vi "Number_2_string.vi"(1 "precision":string, 2 "number":dbl format="%.5f") -> (0 "String":string)   [LabVIEW 2020]
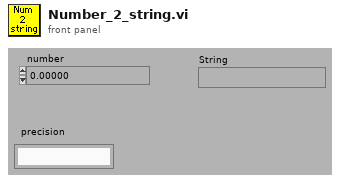
[diagram p1: front panel]
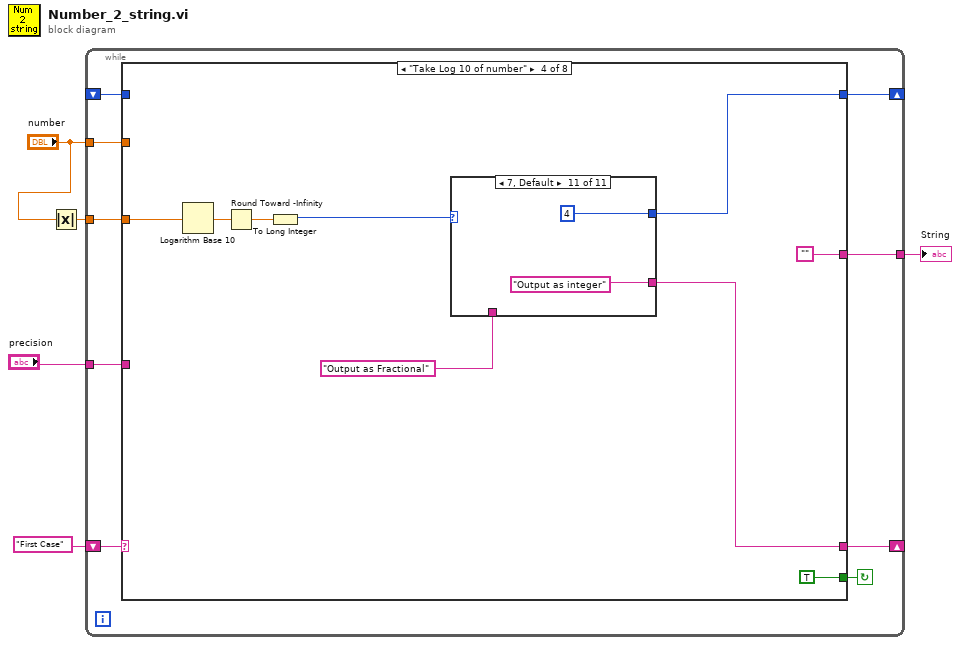
[diagram p0: block diagram]
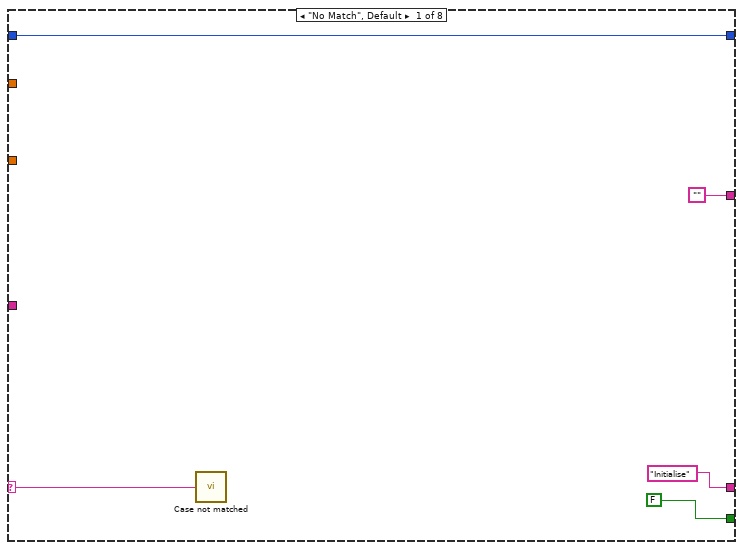
[diagram p2: hidden frame]
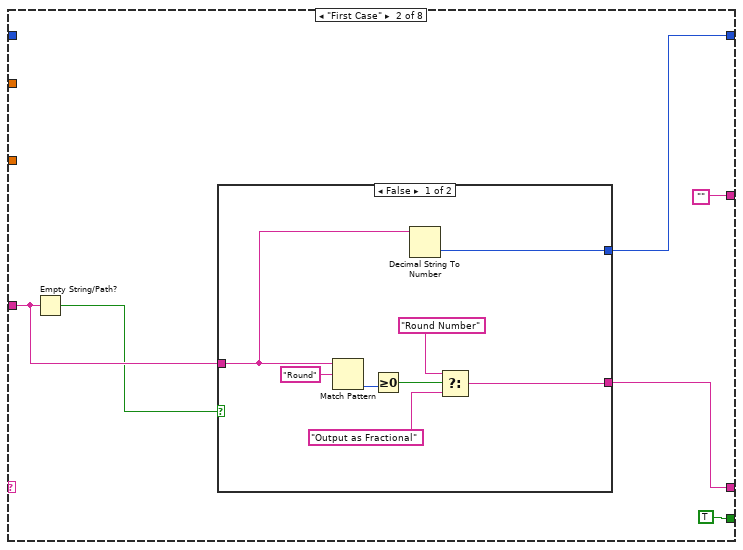
[diagram p3: hidden frame]
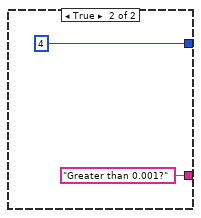
[diagram p4: hidden frame]
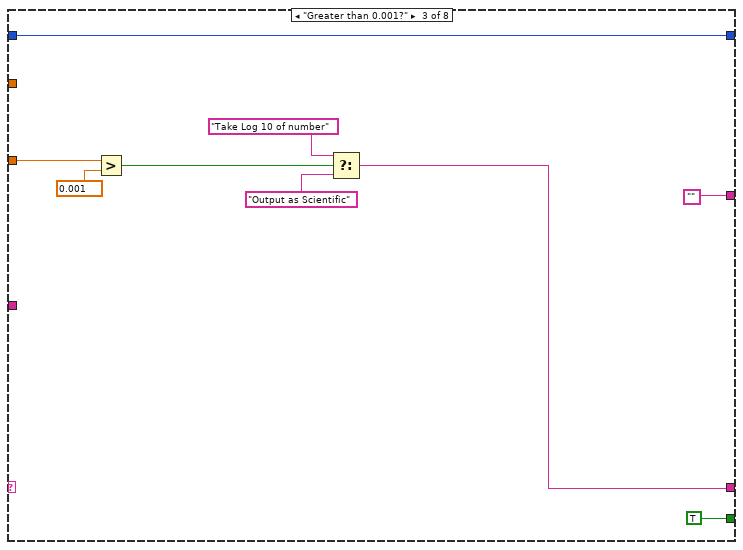
[diagram p5: hidden frame]
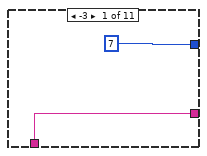
[diagram p6: hidden frame]
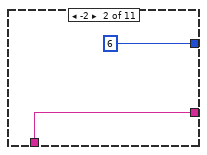
[diagram p7: hidden frame]
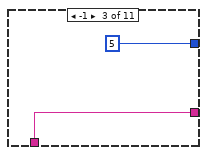
[diagram p8: hidden frame]
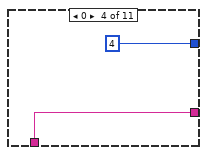
[diagram p9: hidden frame]
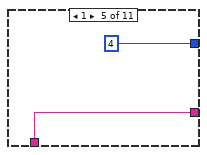
[diagram p10: hidden frame]
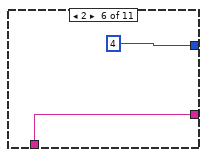
[diagram p11: hidden frame]
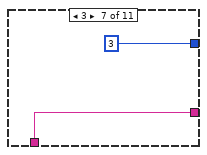
[diagram p12: hidden frame]
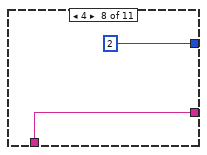
[diagram p13: hidden frame]
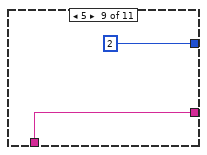
[diagram p14: hidden frame]
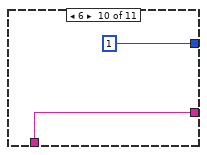
[diagram p15: hidden frame]
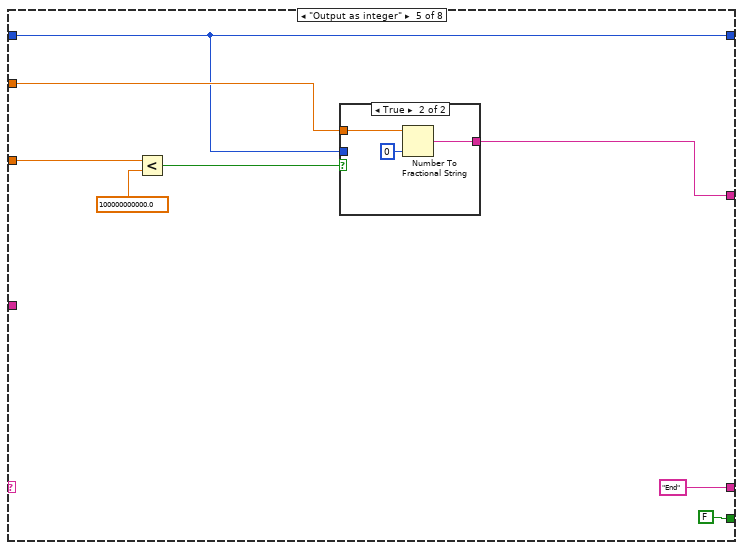
[diagram p16: hidden frame]
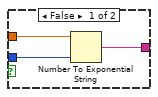
[diagram p17: hidden frame]
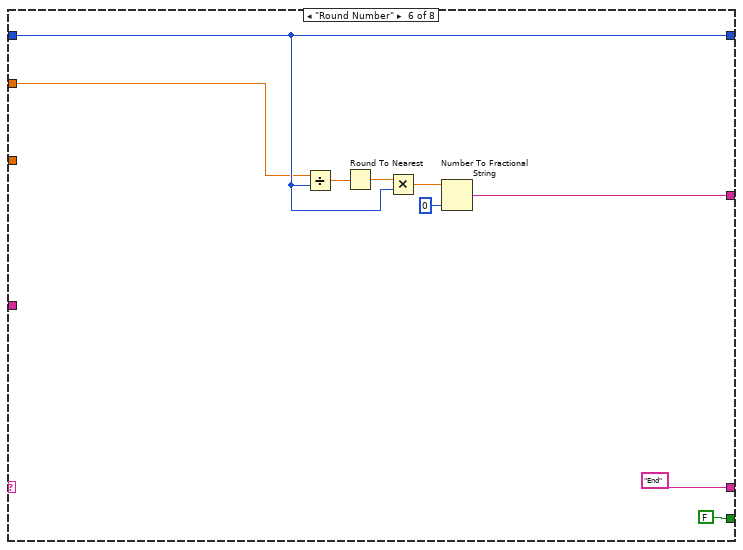
[diagram p18: hidden frame]
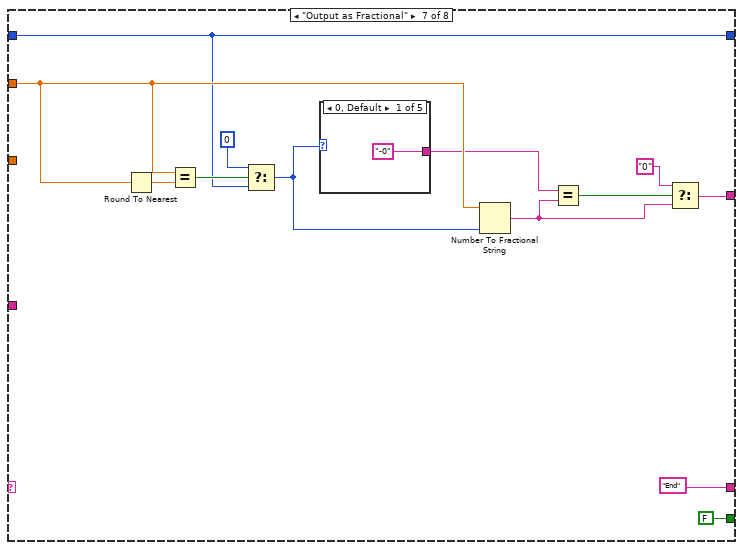
[diagram p19: hidden frame]
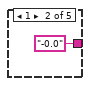
[diagram p20: hidden frame]
diagram:
  n1 = Absolute Value(x="number") -> (abs(x)=w2:dbl)
  n2 = while {
    shift-left: "First Case" -> [w12]
    shift-right: [w13] -> _
    tunnel: "precision" -> [w11]
    tunnel: "number" -> [w10]
    tunnel: w2 -> [w9]
    tunnel: [w8] -> w1
    shift-right: [w7] -> _
    shift-left: _ -> [w6]
    stop <- w14 continue-if-true
    n3 = case shown="\"Take Log 10 of number\"" w12 {
      selector: w12 -> [w15 _ _ _ _ _ _ _]
      tunnel: [FALSE TRUE TRUE TRUE FALSE FALSE FALSE FALSE] -> w14
      tunnel: ["Initialise" w21 w40 w45 "End" "End" "End" "End"] -> w13
      tunnel: w11 -> [_ w24 _ _ _ _ _ _]
      tunnel: w10 -> [_ _ _ _ w78 w90 w108 w118]
      tunnel: w9 -> [_ _ w42 w52 w80 _ _ _]
      tunnel: ["" "" "" "" w77 w91 w104 w120] -> w8
      tunnel: [w16 w22 w36 w48 w76 w94 w101 w119] -> w7
      tunnel: w6 -> [w16 _ w36 _ w76 w94 w101 w119]
      frame "No Match", Default {
        n4 = call "Case not matched.vi"("Case Name not Matched"=w15) -> ()
      }
      frame "First Case" {
        n5 = Empty String/Path?(string/path=w24) -> (empty?=w23:bool)
        n6 = case shown="False" w23 {
          tunnel: w24 -> [w30 _]
          tunnel: [w29 4] -> w22
          tunnel: [w27 "Greater than 0.001?" ("f")] -> w21
          frame False {
            n7 = Match Pattern(string=w30, regular expression="Round") -> (offset past match=w33:i32)  [unwired: 4 out]
            n8 = Greater Or Equal To 0?(x=w33) -> (x >= 0?=w31:bool)
            n9 = Decimal String To Number(string=w30) -> (number=w29:i32)  [unwired: 3 out]
            n10 = Select(t="Round Number", s=w31, f="Output as Fractional") -> (s? t:f=w27:string)
          }
          frame True {
          }
        }
      }
      frame "Greater than 0.001?" {
        n11 = Greater?(x=w42, y=0.001) -> (0:w41:bool)
        n12 = Select(t="Take Log 10 of number", s=w41, f="Output as Scientific") -> (s? t:f=w40:string)
      }
      frame "Take Log 10 of number" {
        n13 = Logarithm Base 10(1:w52) -> (0:w50:dbl)
        n14 = Round Toward -Infinity(1:w50) -> (0:w51:dbl)
        n15 = To Long Integer(number=w51) -> (32bit integer=w49:i32)
        n16 = case shown="7, Default" w49 {
          tunnel: [7 6 5 4 4 4 3 2 2 1 4] -> w48
          tunnel: [w54 w56 w58 w60 w62 w64 w66 w68 w70 w72 "Output as integer"] -> w45
          tunnel: "Output as Fractional" -> [w54 w56 w58 w60 w62 w64 w66 w68 w70 w72 _]
          frame -3 {
          }
          frame -2 {
          }
          frame -1 {
          }
          frame 0 {
          }
          frame 1 {
          }
          frame 2 {
          }
          frame 3 {
          }
          frame 4 {
          }
          frame 5 {
          }
          frame 6 {
          }
          frame 7, Default {
          }
        }
      }
      frame "Output as integer" {
        n17 = Less?(x=w80, y=100000000000.0) -> (x < y?=w79:bool)
        n18 = case shown="True" w79 {
          tunnel: [w85 w89] -> w77
          tunnel: w78 -> [w86 w87]
          tunnel: w76 -> [w84 _]
          frame False {
            n19 = Number To Exponential String(number=w86, precision (6)=w84) -> (E-format string=w85:string)  [unwired: 2 out]
          }
          frame True {
            n20 = Number To Fractional String(number=w87, precision (6)=i16 0) -> (F-format string=w89:string)  [unwired: 2 out]
          }
        }
      }
      frame "Round Number" {
        n21 = Divide(x=w90, y=w94) -> (x/y=w96:dbl)
        n22 = Round To Nearest(number=w96) -> (nearest integer value=w95:dbl)
        n23 = Multiply(x=w95, y=w94) -> (x*y=w93:dbl)
        n24 = Number To Fractional String(number=w93, precision (6)=0) -> (F-format string=w91:string)  [unwired: 2 out]
      }
      frame "Output as Fractional" {
        n25 = Round To Nearest(number=w108) -> (nearest integer value=w109:dbl)
        n26 = Equal?(x=w108, y=w109) -> (x = y?=w103:bool)
        n27 = Select(t=0, s=w103, f=w101) -> (s? t:f=w100:i32)
        n28 = case shown="0, Default" w100 {
          tunnel: ["-0" ("x") "-0.0" ("x") "-0.00" ("x") "-0.000" ("x") "-0.0000" ("x")] -> w99
          frame 0, Default {
          }
          frame 1 {
          }
          frame 2 {
          }
          frame 3 {
          }
          frame 4 {
          }
        }
        n29 = Number To Fractional String(number=w108, precision (6)=w100) -> (F-format string=w106:string)  [unwired: 2 out]
        n30 = Equal?(x=w99, y=w106) -> (x = y?=w107:bool)
        n31 = Select(t="0", s=w107, f=w106) -> (s? t:f=w104:string)
      }
      frame "Output as Scientific" {
        n32 = Equal To 0?(x=w118) -> (x = 0?=w117:bool)
        n33 = case shown="True" w117 {
          tunnel: [w125 "0"] -> w120
          tunnel: w119 -> [w124 _]
          tunnel: w118 -> [w123 _]
          frame False {
            n34 = Number To Exponential String(number=w123, precision (6)=w124) -> (E-format string=w125:string)  [unwired: 2 out]
          }
          frame True {
          }
        }
      }
    }
  }
  "String" <- w1
